vi "Load MPU calib.vi"(8 "Error In":errorcluster, 11 "Calib file path":path) -> (0 "Error Out":errorcluster, 2 "MPU calib data":T1)   [LabVIEW 2016]
uses:
  <vilib>/Utility/config.llb/Read Key (Double).vi
  <vilib>/Utility/config.llb/NI_LVConfig.lvlib
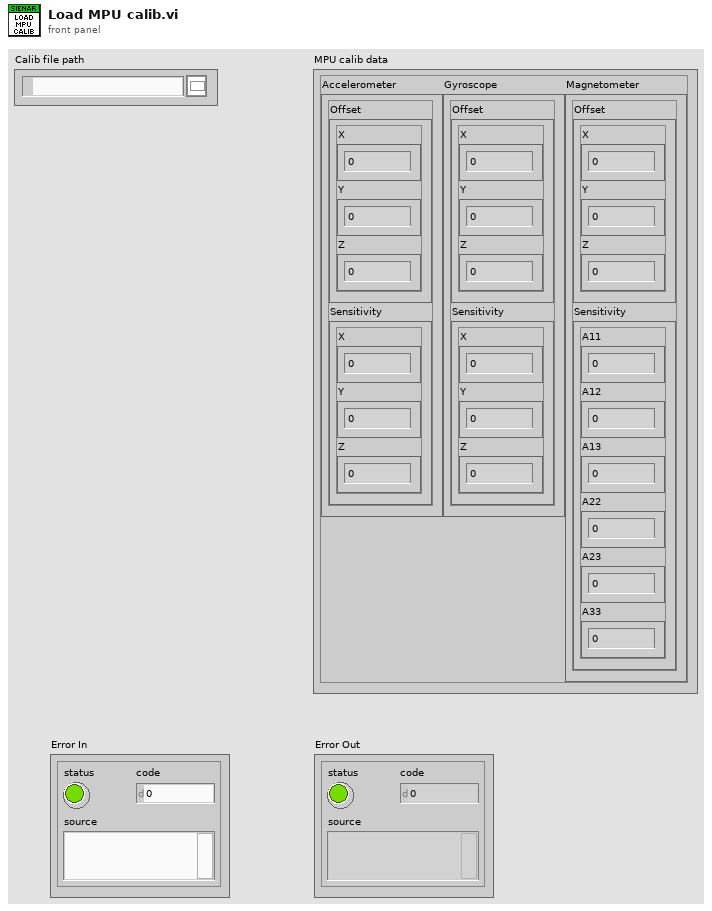
[diagram p1: front panel]
types:
  T1 = cluster{"Accelerometer":cluster{"Offset":cluster{"X":i16, "Y":i16, "Z":i16}, "Sensitivity":cluster{"X":sgl, "Y":sgl, "Z":sgl}}, "Gyroscope":cluster{"Offset":cluster{"X":i16, "Y":i16, "Z":i16}, "Sensitivity":cluster{"X":sgl, "Y":sgl, "Z":sgl}}, "Magnetometer":cluster{"Offset":cluster{"X":i16, "Y":i16, "Z":i16}, "Sensitivity":cluster{"A11":sgl, "A12":sgl, "A13":sgl, "A22":sgl, "A23":sgl, "A33":sgl}}}
  T2 = typedef "NI_LVConfig.lvlib/Config Data RefNum.ctl" = refnum<k1>
  T3 = cluster{cluster{i16, i16, i16}, cluster{sgl, sgl, sgl}}
  T4 = cluster{cluster{i16, i16, i16}, cluster{sgl, sgl, sgl, sgl, sgl, sgl}}
  T5 = cluster{cluster{cluster{i16, i16, i16}, cluster{sgl, sgl, sgl}}, cluster{cluster{i16, i16, i16}, cluster{sgl, sgl, sgl}}, cluster{cluster{i16, i16, i16}, cluster{sgl, sgl, sgl, sgl, sgl, sgl}}}
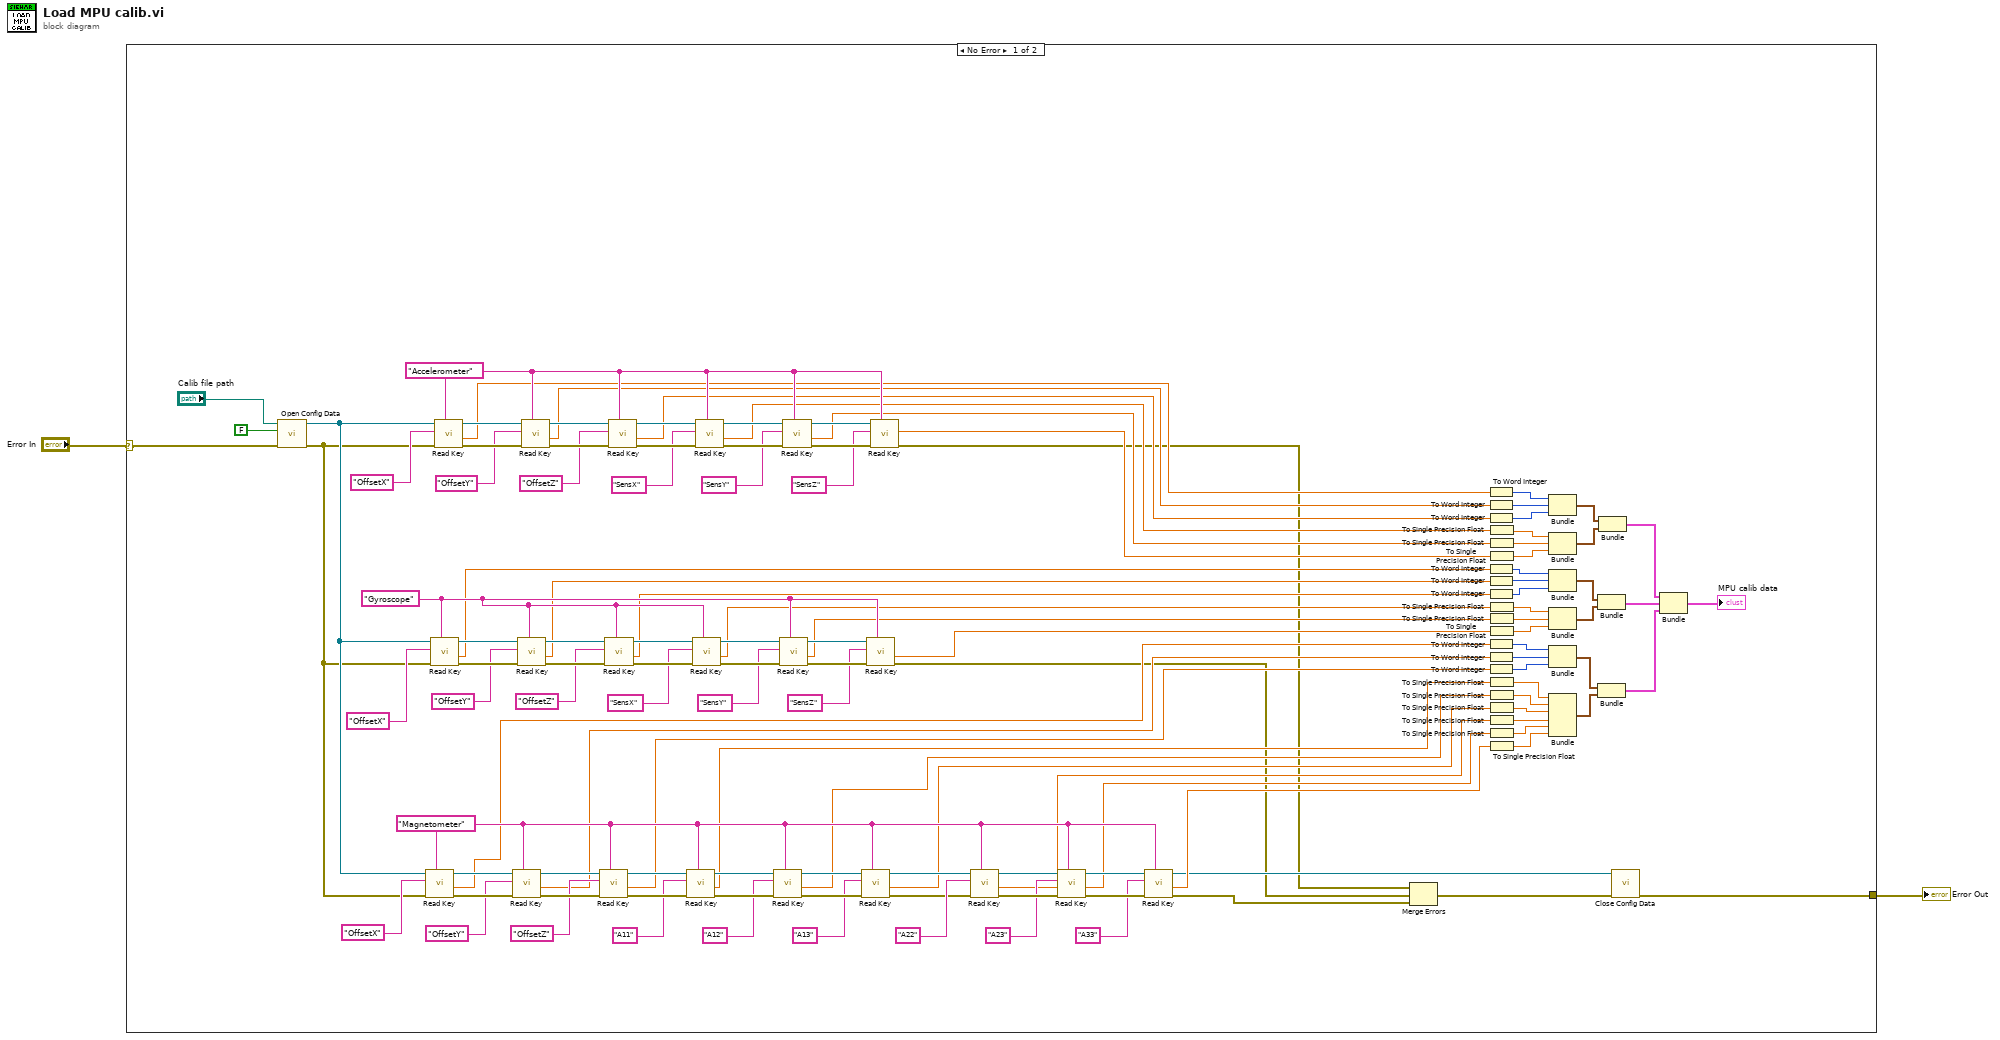
[diagram p0: block diagram]
diagram:
  n1 = case shown="No Error" "Error In" {
    selector: "Error In" -> [w124 w126]
    tunnel: [w125 w126] -> w2
    frame No Error {
      w60 = "Magnetometer" ("section")
      w104 = "Gyroscope" ("section")
      w121 = "Accelerometer" ("section")
      n2 = call <vilib>:"Open Config Data.vi"("error in (no error)"=w124, "create file if necessary (T)"=FALSE, "configuration file path"="Calib file path") -> ("error out"=w70:errorcluster, "refnum"=w71:T2)  [unwired: 6 in, 1 out]
      n3 = call-poly <vilib>:"Read Key.vi"("section"=w60, "error in (no error)"=w70, "key"="OffsetX", "refnum"=w71) -> ("error out"=w87:errorcluster, "value"=w47:dbl, "refnum out"=w82:T2)  [unwired: 4 in, 1 out]
      n4 = call-poly <vilib>:"Read Key.vi"("section"=w104, "error in (no error)"=w70, "key"="OffsetX", "refnum"=w71) -> ("error out"=w103:errorcluster, "value"=w53:dbl, "refnum out"=w98:T2)  [unwired: 4 in, 1 out]
      n5 = call-poly <vilib>:"Read Key.vi"("section"=w121, "error in (no error)"=w70, "key"="OffsetX", "refnum"=w71) -> ("error out"=w120:errorcluster, "value"=w59:dbl, "refnum out"=w115:T2)  [unwired: 4 in, 1 out]
      n6 = call-poly <vilib>:"Read Key.vi"("section"=w60, "error in (no error)"=w87, "key"="OffsetY", "refnum"=w82) -> ("error out"=w86:errorcluster, "value"=w46:dbl, "refnum out"=w81:T2)  [unwired: 4 in, 1 out]
      n7 = call-poly <vilib>:"Read Key.vi"("section"=w104, "error in (no error)"=w103, "key"="OffsetY", "refnum"=w98) -> ("error out"=w102:errorcluster, "value"=w52:dbl, "refnum out"=w97:T2)  [unwired: 4 in, 1 out]
      n8 = call-poly <vilib>:"Read Key.vi"("section"=w121, "error in (no error)"=w120, "key"="OffsetY", "refnum"=w115) -> ("error out"=w119:errorcluster, "value"=w58:dbl, "refnum out"=w114:T2)  [unwired: 4 in, 1 out]
      n9 = call-poly <vilib>:"Read Key.vi"("section"=w60, "error in (no error)"=w86, "key"="OffsetZ", "refnum"=w81) -> ("error out"=w85:errorcluster, "value"=w45:dbl, "refnum out"=w80:T2)  [unwired: 4 in, 1 out]
      n10 = call-poly <vilib>:"Read Key.vi"("section"=w104, "error in (no error)"=w102, "key"="OffsetZ", "refnum"=w97) -> ("error out"=w101:errorcluster, "value"=w51:dbl, "refnum out"=w96:T2)  [unwired: 4 in, 1 out]
      n11 = call-poly <vilib>:"Read Key.vi"("section"=w121, "error in (no error)"=w119, "key"="OffsetZ", "refnum"=w114) -> ("error out"=w118:errorcluster, "value"=w57:dbl, "refnum out"=w113:T2)  [unwired: 4 in, 1 out]
      n12 = call-poly <vilib>:"Read Key.vi"("section"=w60, "error in (no error)"=w85, "key"="A11", "refnum"=w80) -> ("error out"=w84:errorcluster, "value"=w44:dbl, "refnum out"=w79:T2)  [unwired: 4 in, 1 out]
      n13 = call-poly <vilib>:"Read Key.vi"("section"=w104, "error in (no error)"=w101, "key"="SensX", "refnum"=w96) -> ("error out"=w100:errorcluster, "value"=w50:dbl, "refnum out"=w95:T2)  [unwired: 4 in, 1 out]
      n14 = call-poly <vilib>:"Read Key.vi"("section"=w121, "error in (no error)"=w118, "key"="SensX", "refnum"=w113) -> ("error out"=w117:errorcluster, "value"=w56:dbl, "refnum out"=w112:T2)  [unwired: 4 in, 1 out]
      n15 = call-poly <vilib>:"Read Key.vi"("section"=w60, "error in (no error)"=w84, "key"="A12", "refnum"=w79) -> ("error out"=w83:errorcluster, "value"=w43:dbl, "refnum out"=w78:T2)  [unwired: 4 in, 1 out]
      n16 = call-poly <vilib>:"Read Key.vi"("section"=w104, "error in (no error)"=w100, "key"="SensY", "refnum"=w95) -> ("error out"=w99:errorcluster, "value"=w49:dbl, "refnum out"=w94:T2)  [unwired: 4 in, 1 out]
      n17 = call-poly <vilib>:"Read Key.vi"("section"=w121, "error in (no error)"=w117, "key"="SensY", "refnum"=w112) -> ("error out"=w116:errorcluster, "value"=w55:dbl, "refnum out"=w111:T2)  [unwired: 4 in, 1 out]
      n18 = call-poly <vilib>:"Read Key.vi"("section"=w60, "error in (no error)"=w83, "key"="A13", "refnum"=w78) -> ("error out"=w61:errorcluster, "value"=w42:dbl, "refnum out"=w62:T2)  [unwired: 4 in, 1 out]
      n19 = call-poly <vilib>:"Read Key.vi"("section"=w104, "error in (no error)"=w99, "key"="SensZ", "refnum"=w94) -> ("error out"=w35:errorcluster, "value"=w48:dbl)  [unwired: 4 in, 2 out]
      n20 = call-poly <vilib>:"Read Key.vi"("section"=w121, "error in (no error)"=w116, "key"="SensZ", "refnum"=w111) -> ("error out"=w34:errorcluster, "value"=w54:dbl)  [unwired: 4 in, 2 out]
      n21 = call-poly <vilib>:"Read Key.vi"("section"=w60, "error in (no error)"=w61, "key"="A22", "refnum"=w62) -> ("error out"=w69:errorcluster, "value"=w41:dbl, "refnum out"=w67:T2)  [unwired: 4 in, 1 out]
      n22 = call-poly <vilib>:"Read Key.vi"("section"=w60, "error in (no error)"=w69, "key"="A23", "refnum"=w67) -> ("error out"=w68:errorcluster, "value"=w40:dbl, "refnum out"=w66:T2)  [unwired: 4 in, 1 out]
      n23 = call-poly <vilib>:"Read Key.vi"("section"=w60, "error in (no error)"=w68, "key"="A33", "refnum"=w66) -> ("error out"=w37:errorcluster, "value"=w39:dbl, "refnum out"=w38:T2)  [unwired: 4 in, 1 out]
      n24 = Merge Errors(w34, w35, w37) -> (w36:errorcluster)
      n25 = To Word Integer(number=w59) -> (16bit integer=w33:i16)
      n26 = To Word Integer(number=w58) -> (16bit integer=w32:i16)
      n27 = To Word Integer(number=w57) -> (16bit integer=w31:i16)
      n28 = To Word Integer(number=w53) -> (16bit integer=w27:i16)
      n29 = To Word Integer(number=w52) -> (16bit integer=w26:i16)
      n30 = To Word Integer(number=w51) -> (16bit integer=w25:i16)
      n31 = To Word Integer(number=w47) -> (16bit integer=w21:i16)
      n32 = To Word Integer(number=w46) -> (16bit integer=w20:i16)
      n33 = To Word Integer(number=w45) -> (16bit integer=w19:i16)
      n34 = To Single Precision Float(number=w56) -> (single precision float=w30:sgl)
      n35 = To Single Precision Float(number=w55) -> (single precision float=w29:sgl)
      n36 = To Single Precision Float(number=w54) -> (single precision float=w28:sgl)
      n37 = To Single Precision Float(number=w50) -> (single precision float=w24:sgl)
      n38 = To Single Precision Float(number=w49) -> (single precision float=w23:sgl)
      n39 = To Single Precision Float(number=w48) -> (single precision float=w22:sgl)
      n40 = To Single Precision Float(number=w44) -> (single precision float=w18:sgl)
      n41 = To Single Precision Float(number=w43) -> (single precision float=w17:sgl)
      n42 = To Single Precision Float(number=w42) -> (single precision float=w16:sgl)
      n43 = To Single Precision Float(number=w41) -> (single precision float=w15:sgl)
      n44 = To Single Precision Float(number=w40) -> (single precision float=w14:sgl)
      n45 = To Single Precision Float(number=w39) -> (single precision float=w13:sgl)
      n46 = Bundle(w33, w32, w31) -> (w12:cluster{i16, i16, i16})  [unwired: 1 in]
      n47 = Bundle(w30, w29, w28) -> (w11:cluster{sgl, sgl, sgl})  [unwired: 1 in]
      n48 = Bundle(w27, w26, w25) -> (w10:cluster{i16, i16, i16})  [unwired: 1 in]
      n49 = Bundle(w24, w23, w22) -> (w9:cluster{sgl, sgl, sgl})  [unwired: 1 in]
      n50 = Bundle(w21, w20, w19) -> (w8:cluster{i16, i16, i16})  [unwired: 1 in]
      n51 = Bundle(w18, w17, w16, w15, w14, w13) -> (w7:cluster{sgl, sgl, sgl, sgl, sgl, sgl})  [unwired: 1 in]
      n52 = Bundle(w10, w9) -> (w5:T3)  [unwired: 1 in]
      n53 = Bundle(w8, w7) -> (w4:T4)  [unwired: 1 in]
      n54 = Bundle(w12, w11) -> (w6:T3)  [unwired: 1 in]
      n55 = call <vilib>:"Close Config Data.vi"("error in (no error)"=w36, "refnum"=w38) -> ("error out"=w125:errorcluster)  [unwired: 8 in, 1 out]
      n56 = Bundle(w6, w5, w4) -> (→"MPU calib data":T5)  [unwired: 1 in]
    }
    frame Error {
    }
  }
  "Error Out" <- w2
